vi "pickDefensivePlay.vi"(8 "error in (no error)":errorcluster, 11 "Game in":refnum<class "Game.lvclass">) -> (0 "error out":errorcluster, 3 "Game out":refnum<class "Game.lvclass">)   [LabVIEW 2018, in "Game.lvclass"]
uses:
  Game.lvclass
  Team_class/DefensivePlay.ctl
  Game.lvclass/Game.ctl
  Team_class/Team.lvclass/Team.ctl
  Read AllyRef.vi
  Team_class/Write DefensivePlay.vi
  Write AllyRef.vi
  Ally_class/Ally.lvclass
  C:/Users/nicolas.oliveira/roboime/SSL_AI/Team_class/Team.lvclass
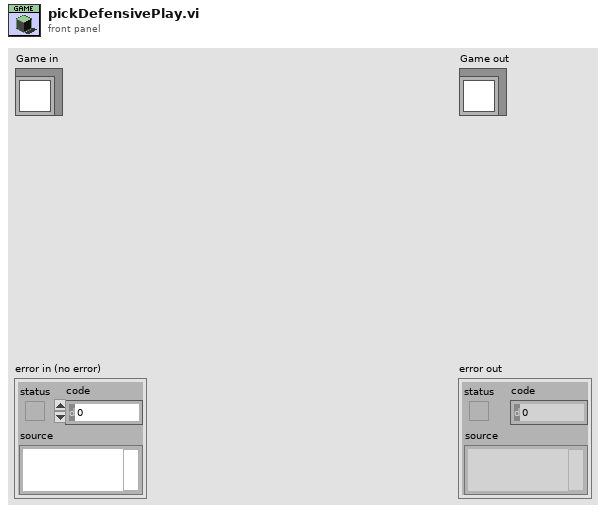
[diagram p1: front panel]
types:
  T1 = typedef "DefensivePlay.ctl" = enum16{"TestPlay", "Default", "Duelist", "Halt", "Timeout", "PenaltyEnemy", "PenaltyAlly"}
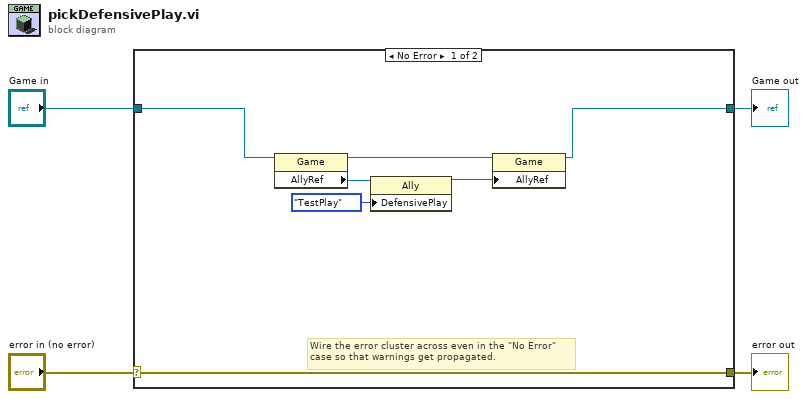
[diagram p0: block diagram]
diagram:
  n1 = case shown="No Error" "error in (no error)" {
    selector: "error in (no error)" -> [w11 w13]
    tunnel: [w11 w13] -> w3
    tunnel: [w5 w12] -> w1
    tunnel: "Game in" -> [w6 w12]
    frame No Error {
      # "Wire the error cluster across even in the \"No Error\"\ncase so that warnings get propagated."
      n2 = property class="Game"(reference=w6) -> (reference out=w9:refnum<class "Game.lvclass">, "AllyRef"=w10:refnum<class "Ally.lvclass">)  [unwired: 1 in, 1 out]
      n3 = property class="Ally"(reference=w10, "DefensivePlay"=DefensivePlay."TestPlay") -> (reference out=w8:refnum<class "Ally.lvclass">)  [unwired: 1 in, 1 out]
      n4 = property class="Game"(reference=w9, "AllyRef"=w8) -> (reference out=w5:refnum<class "Game.lvclass">)  [unwired: 1 in, 1 out]
    }
    frame Error {
    }
  }
  "error out" <- w3
  "Game out" <- w1
